vi "Number of Tabs - Minimum--Const.vi"() -> (3 "Minimum Tabs":i32)   [LabVIEW 2017, in "DTacq Plot Display Library.lvlib"]
uses:
  DTacq Plot Display Library.lvlib
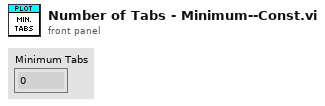
[diagram p1: front panel]
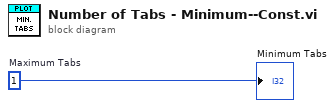
[diagram p0: block diagram]
diagram:
  w1 = 1  # Maximum Tabs
  "Minimum Tabs" <- w1
